vi "Day 9-Compute Basin Sizes using Sets.vi"(10 "Padded Data Array in":i32[][](array[numeric]), 11 "Low Point Coordinates":i32[][](array[numeric])) -> (3 "All Basin Sizes":i32[](array[numeric]))   [LabVIEW 2021]
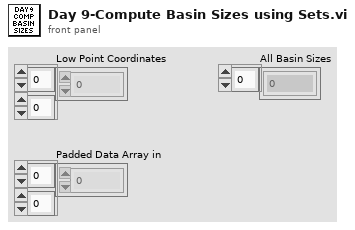
[diagram p1: front panel]
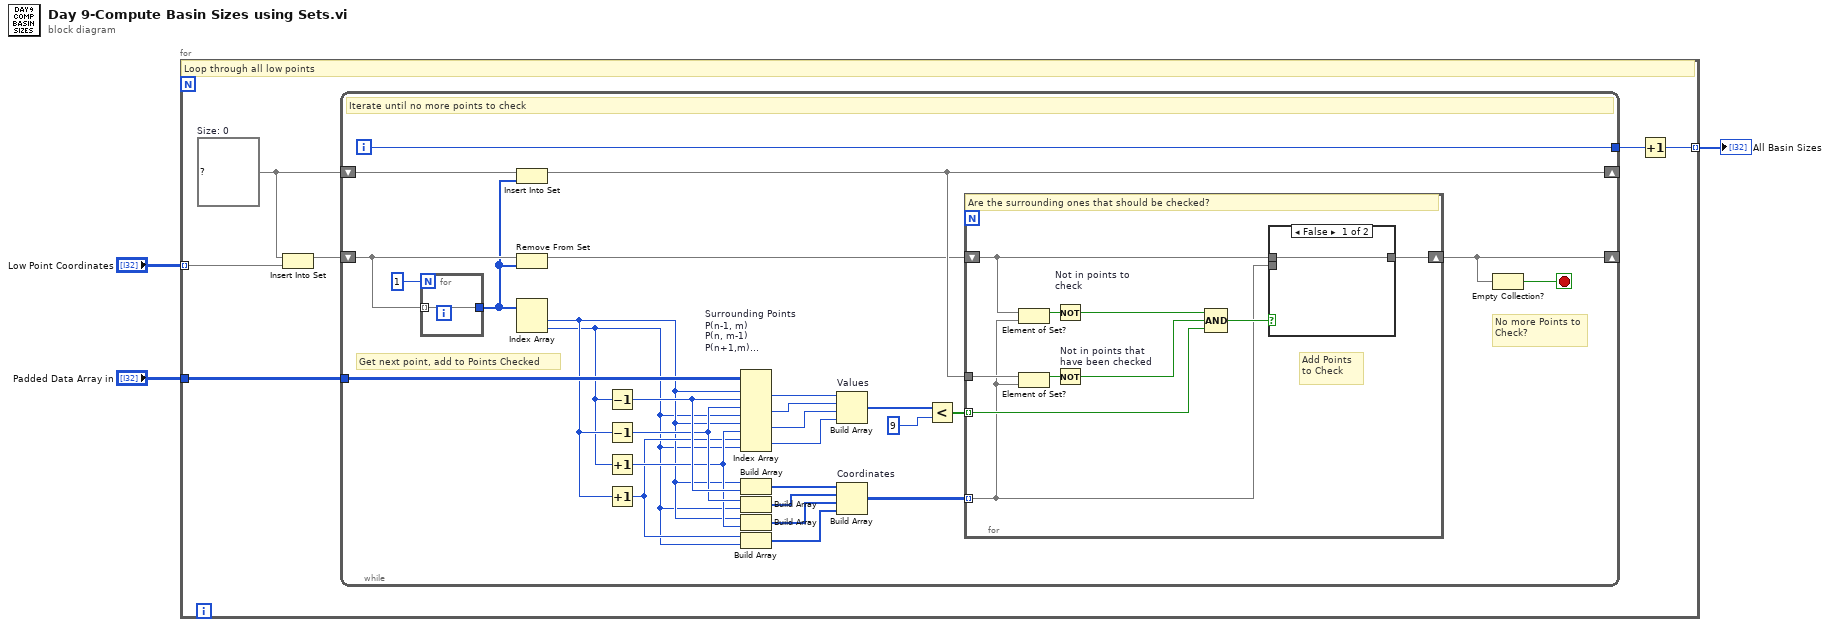
[diagram p0: block diagram]
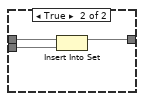
[diagram p2: hidden frame]
diagram:
  n1 = for {
    tunnel: "Low Point Coordinates" -> [w4] mode=indexing
    tunnel: [w8] -> w1 mode=indexing
    tunnel: "Padded Data Array in" -> [w7]
    w6 = set{i32[]} {}  # Size: 0
    # "Loop through all low points"
    n2 = Insert Into Set(10:w4, 11:w6) -> (3:w5:set{i32[]})  [unwired: 1 out]
    n3 = while {
      shift-right: [w11] -> _
      shift-left: w5 -> [w14]
      tunnel: w7 -> [w37]
      tunnel: [w18] -> w9
      shift-right: [w16] -> _
      shift-left: w6 -> [w17]
      i -> [w18]
      stop <- w10 stop-if-true
      # "Get next point, add to Points Checked"
      # "No more Points to Check?"
      # "Iterate until no more points to check"
      n4 = for {
        N: 1 -> [_]
        tunnel: w14 -> [w38] mode=indexing
        tunnel: [w38] -> w13
      }
      n5 = Insert Into Set(10:w13, 11:w17) -> (3:w16:set{i32[]})  [unwired: 1 out]
      n6 = Remove From Set(10:w13, 11:w14) -> (3:w12:set{i32[]})  [unwired: 1 out]
      n7 = Index Array(array=w13) -> (element #1=w20:i32, element #2=w19:i32)  [unwired: 2 in]
      n8 = Decrement(x=w19) -> (x-1=w30:i32)
      n9 = Decrement(x=w20) -> (x-1=w29:i32)
      n10 = Increment(x=w19) -> (x+1=w28:i32)
      n11 = Increment(x=w20) -> (x+1=w27:i32)
      n12 = Index Array "Surrounding Points\nP(n-1, m)\nP(n, m-1)\nP(n+1,m)\nP(n, m+1)"(array=w37, index (row) #1=w20, index (col) #1=w30, index (row) #2=w29, index (col) #2=w19, index (row) #3=w20, index (col) #3=w28, index (row) #4=w27, index (col) #4=w19) -> (element #1=w36:i32, element #2=w35:i32, element #3=w34:i32, element #4=w33:i32)
      n13 = Build Array(w20, w30) -> (w26:i32[])
      n14 = Build Array(w29, w19) -> (w25:i32[])
      n15 = Build Array(w20, w28) -> (w24:i32[])
      n16 = Build Array(w27, w19) -> (w23:i32[])
      n17 = Build Array "Values"(w36, w35, w34, w33) -> (w32:i32[])
      n18 = Build Array "Coordinates"(w26, w25, w24, w23) -> (w21:i32[][])
      n19 = Less?(x=w32, y=9) -> (x < y?=w22:bool[])
      n20 = for {
        tunnel: w22 -> [w47] mode=indexing
        tunnel: w21 -> [w40] mode=indexing
        tunnel: w16 -> [w45]
        shift-right: [w42] -> w11
        shift-left: w12 -> [w41]
        # "Add Points to Check"
        # "Are the surrounding ones that should be checked?"
        n21 = Element of Set?(10:w40, 11:w41) -> (3:w39:bool)
        n22 = Element of Set?(10:w40, 11:w45) -> (3:w44:bool)
        n23 = Not "Not in points to\ncheck"(x=w39) -> (.not. x?=w46:bool)
        n24 = Not "Not in points that\nhave been checked"(x=w44) -> (.not. x?=w48:bool)
        n25 = Compound Arithmetic op=AND(w46, w48, w47) -> (w43:bool)
        n26 = case shown="False" w43 {
          tunnel: w41 -> [w49 w52]
          tunnel: w40 -> [_ w51]
          tunnel: [w49 w50] -> w42
          frame False {
          }
          frame True {
            n27 = Insert Into Set(10:w51, 11:w52) -> (3:w50:set{i32[]})  [unwired: 1 out]
          }
        }
      }
      n28 = Empty Collection?(1:w11) -> (0:w10:bool)
    }
    n29 = Increment(x=w9) -> (x+1=w8:i32)
  }
  "All Basin Sizes" <- w1
